vi "picture.publish.vi"(8 "error in":errorcluster, 11 "midi-ui in":refnum<class "midi-ui.lvclass">) -> (0 "error out":errorcluster, 3 "midi-ui out":refnum<class "midi-ui.lvclass">)   [LabVIEW 2020, in "midi-ui.lvclass"]
uses:
  midi-ui.lvclass
  midi-ui.lvclass/midi-ui.ctl
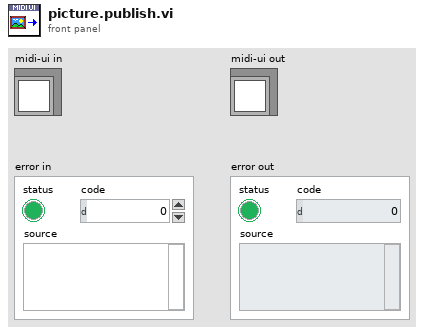
[diagram p1: front panel]
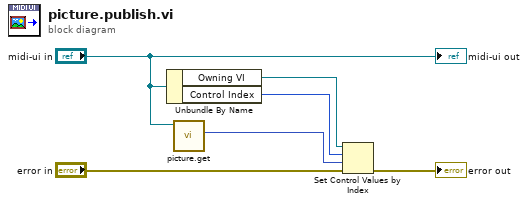
[diagram p0: block diagram]
diagram:
  n1 = Unbundle By Name("midi-ui in") -> ("Owning VI"=w3:refnum<vi>, "Control Index"=w6:i32)
  n2 = call "picture.get.vi"("midi-ui in"="midi-ui in") -> ("image"=w1:picture)  [unwired: 10 in]
  n3 = Set Control Values by Index(0:w3, 1:w6, 2:w1, 3:"error in") -> (11:→"error out":errorcluster)
  "midi-ui out" <- "midi-ui in"
